vi "hmi_browse_post_install_file.vi"(8 "error in (no error)":errorcluster, 11 "post_installer_file":string) -> (0 "error out":errorcluster, 3 "selected path":path)   [LabVIEW 2015, in "lv-builder-default.lvlib"]
uses:
  lv-builder-default.lvlib
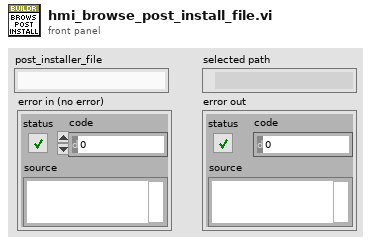
[diagram p1: front panel]
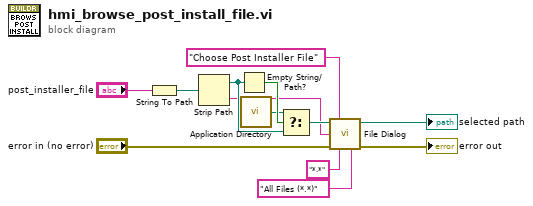
[diagram p0: block diagram]
diagram:
  n1 = String To Path(string="post_installer_file") -> (path=w9:path)
  n2 = Strip Path(path=w9) -> (stripped path=w3:path, name=w1:string)
  n3 = Empty String/Path?(string/path=w3) -> (empty?=w10:bool)
  n4 = call <vilib>:"Application Directory.vi"() -> ("Application Directory"=w7:path)
  n5 = Select(t=w7, s=w10, f=w3) -> (s? t:f=w11:path)
  n6 = call "File Dialog"("start path"=w11, "prompt"="Choose Post Installer File" ("description"), "default name"=w1, "error in"="error in (no error)", "pattern (all files)"="*.*" ("filter"), "pattern label"="All Files (*.*)" ("filter")) -> ("selected path"=→"selected path":path, "error out"=→"error out":errorcluster)  [unwired: 6 in, 2 out]
